vi "Wrapper_getWavelengths.vi"(2 "Index":i32, 3 "Wrapper":u32) -> (0 "Length":i32, 1 "WL Values":dbl[](array[numeric]))   [LabVIEW 2017]
uses:
  common32.dll
  OmniDriver32.dll
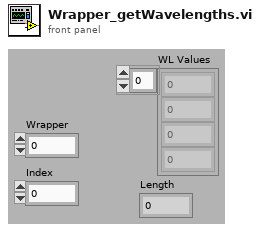
[diagram p1: front panel]
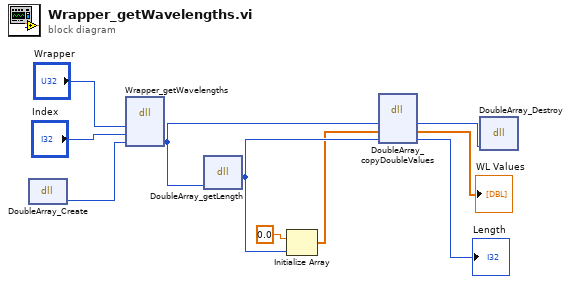
[diagram p0: block diagram]
diagram:
  n1 = dll-call lib="common32.dll" fn="DoubleArray_Create" label="DoubleArray.Create"() -> ("return type"=w8:u32)  [unwired: 3 in, 2 out]
  n2 = dll-call lib="OmniDriver32.dll" fn="Wrapper_getWavelengths" label="Wrapper.getWavelengths"("Wrapper"="Wrapper", "Index"="Index", "WL DoubleArray"=w8) -> ("WL DoubleArray"=w4:u32)  [unwired: 5 in, 3 out]
  n3 = dll-call lib="common32.dll" fn="DoubleArray_getLength" label="DoubleArray.getLength"("DoubbleArray"=w4) -> ("return type"=w6:i32)  [unwired: 4 in, 2 out]
  n4 = Initialize Array(0.0 ("element"), w6) -> (w5:dbl[])
  n5 = dll-call lib="common32.dll" fn="DoubleArray_copyDoubleValues" label="DoubleArray.coopyDoubleValues"("DoubleArray"=w4, "Values"=w5, "Length"=w6) -> ("DoubleArray"=w1:u32, "Values"=→"WL Values":dbl[], "Length"=→"Length":i32)  [unwired: 3 in, 3 out]
  n6 = dll-call lib="common32.dll" fn="DoubleArray_Destroy" label="DoubleArray.Destroy"("DoubleArray"=w1) -> ()  [unwired: 4 in, 3 out]
